vi "Core.vi"() -> (19 "Error Out":errorcluster)   [LabVIEW 2017]
uses:
  <vilib>/Platform/TimedLoop/XDataNode/timing_clust.ctl
  <vilib>/Platform/TimedLoop/XDataNode/nitl_modes.ctl
  <vilib>/Platform/TimedLoop/XDataNode/wakeup.ctl
  <vilib>/Platform/TimedLoop/XDataNode/XDataNode.xnode
  <vilib>/Platform/TimedLoop/XDataNode/XDNodeRunTimeDep.lvlib
panel:
  out "Output Resistance 2":dbl
  in  "Shutdown":bool
  out "Output Resistance":dbl
  # "Core Module DIagnostics"
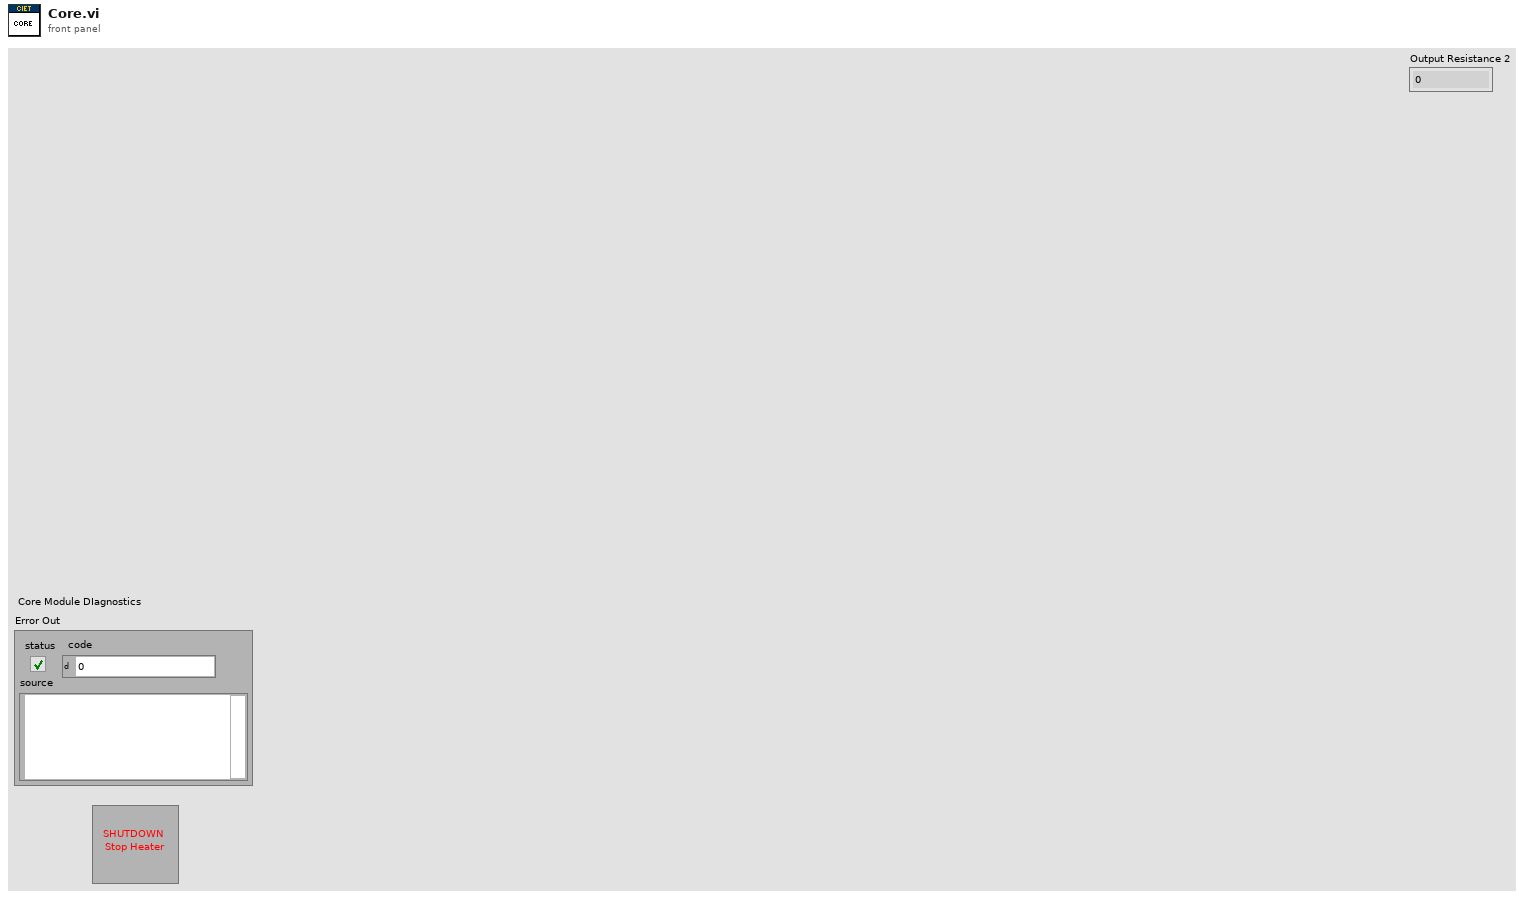
[diagram p1: front panel]
types:
  T1 = typedef "XDNodeRunTimeDep.lvlib/timing_clust.ctl" = cluster{"Expected End [f-1]":u64, "Actual End [f-1]":u64, "Finished Late? [f-1]":bool, "Expected End [i-1]":u64, "Actual End [i-1]":u64, "Finished Late? [i-1]":bool, "Expected Start [i]":u64, "Actual Start [i]":u64, "Expected Start [f]":u64, "Actual Start [f]":u64, "Source Name":string, "Structure Name":string, "Period":i64, "Deadline":i64, "Offset":i64, "Start":i64, "Priority":i32, "Timeout":i32, "Mode":T2, "Wakeup Reason":T3, "Error":errorcluster, "Source Type":string, "Secondary Source Type":string, "Global End Time":u64, "Global Start Time":u64, "Frame Duration":u64, "Iteration Duration":u64, "Assigned CPU":i32, "I/O Scan Engine Mode":u32}
  T2 = typedef "XDNodeRunTimeDep.lvlib/nitl_modes.ctl" = enum32{"No Change", "Process missed periods, maintain original phase", "Discard missed periods, maintain original phase", "Process missed periods, ignore original phase", "Discard missed periods, ignore original phase"}
  T3 = typedef "XDNodeRunTimeDep.lvlib/wakeup.ctl" = enum32{"Normal", "Aborted", "Asynchronous wakeup", "Timing source error", "Timed loop error", "Timeout"}
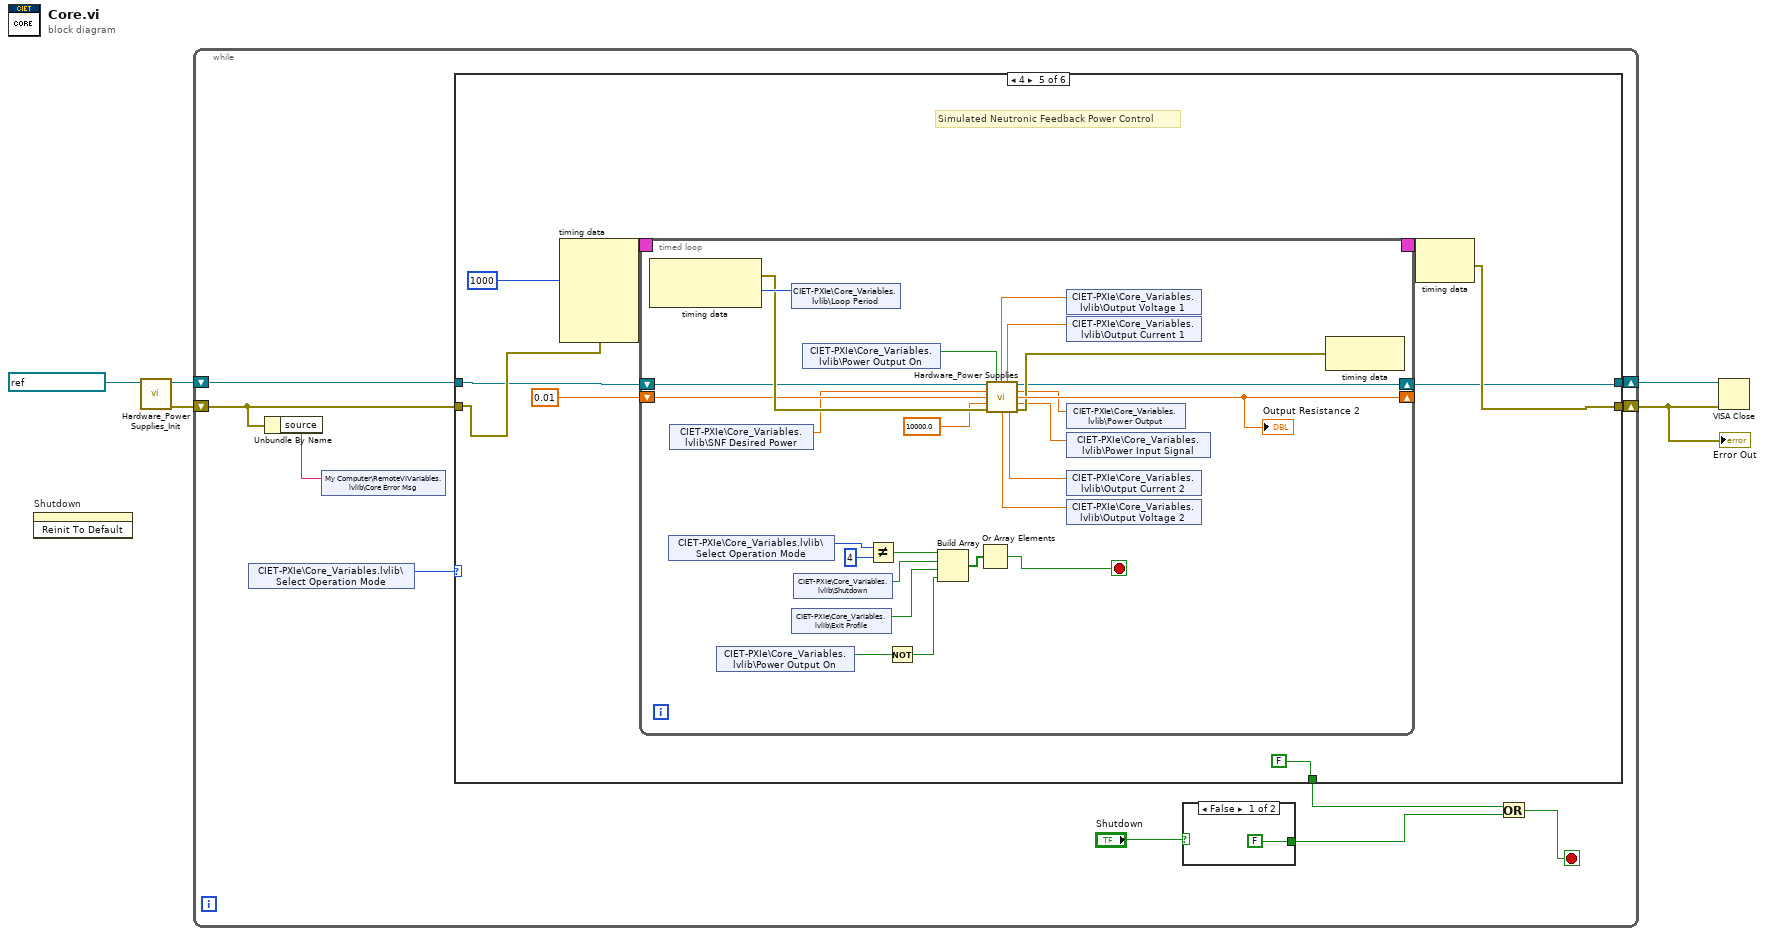
[diagram p0: block diagram]
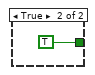
[diagram p2: hidden frame]
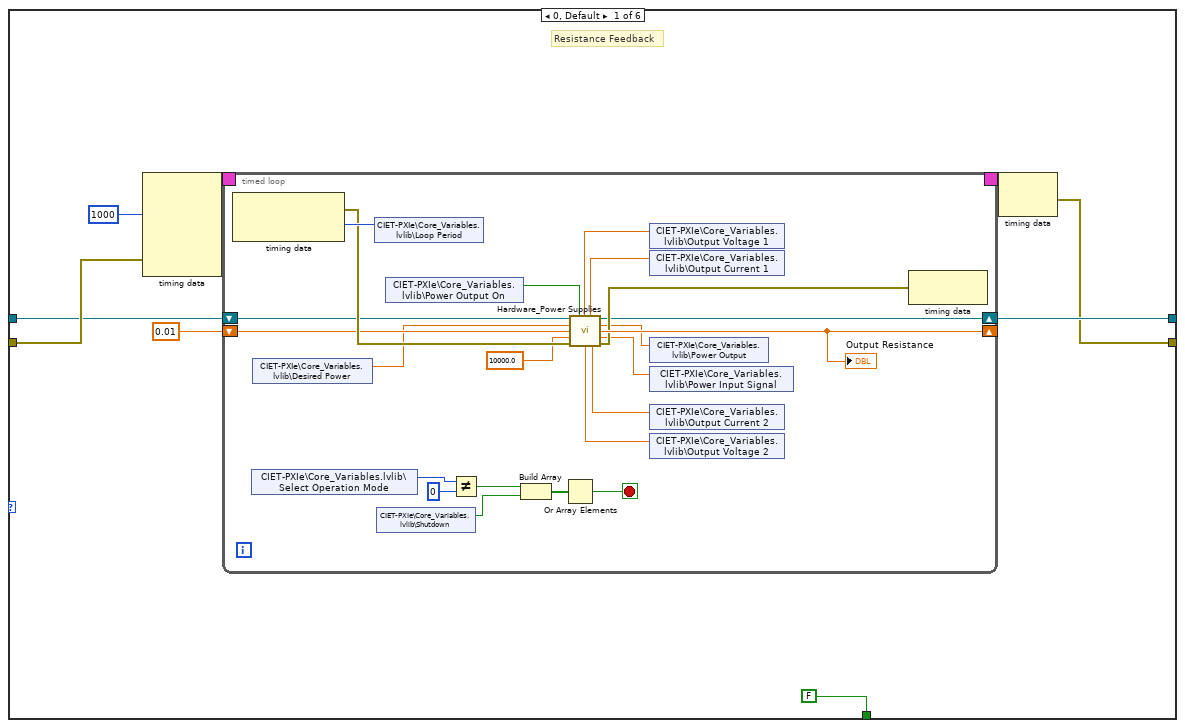
[diagram p3: hidden frame]
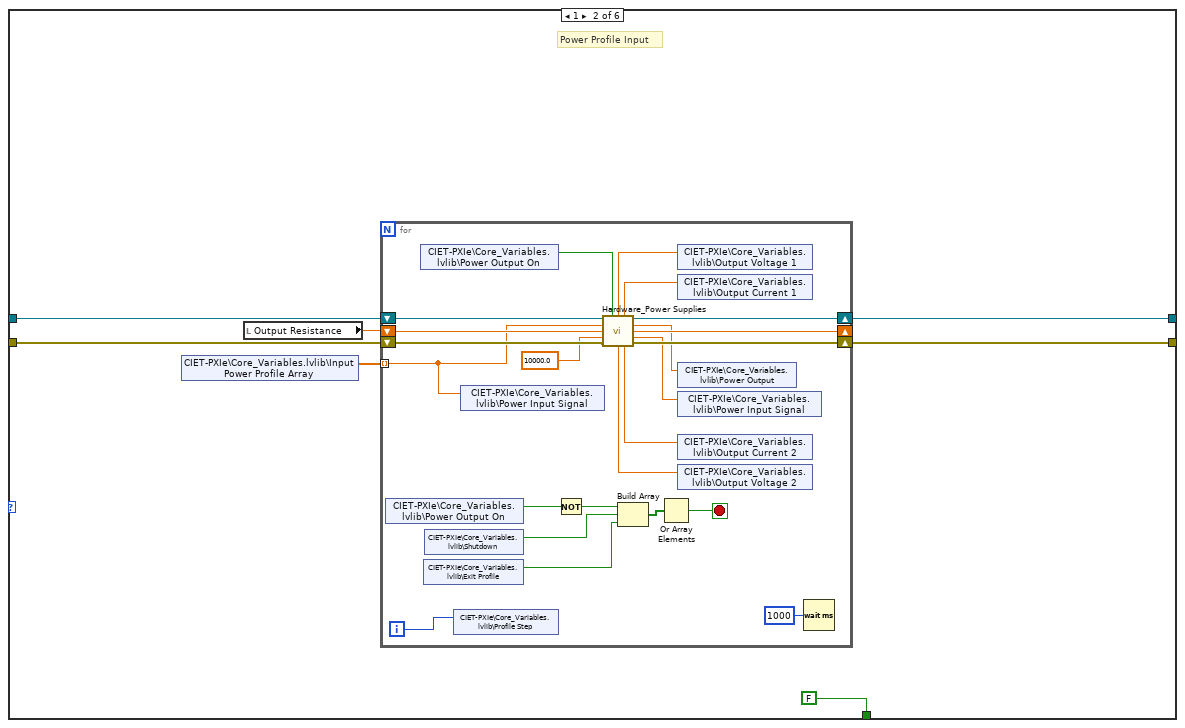
[diagram p4: hidden frame]
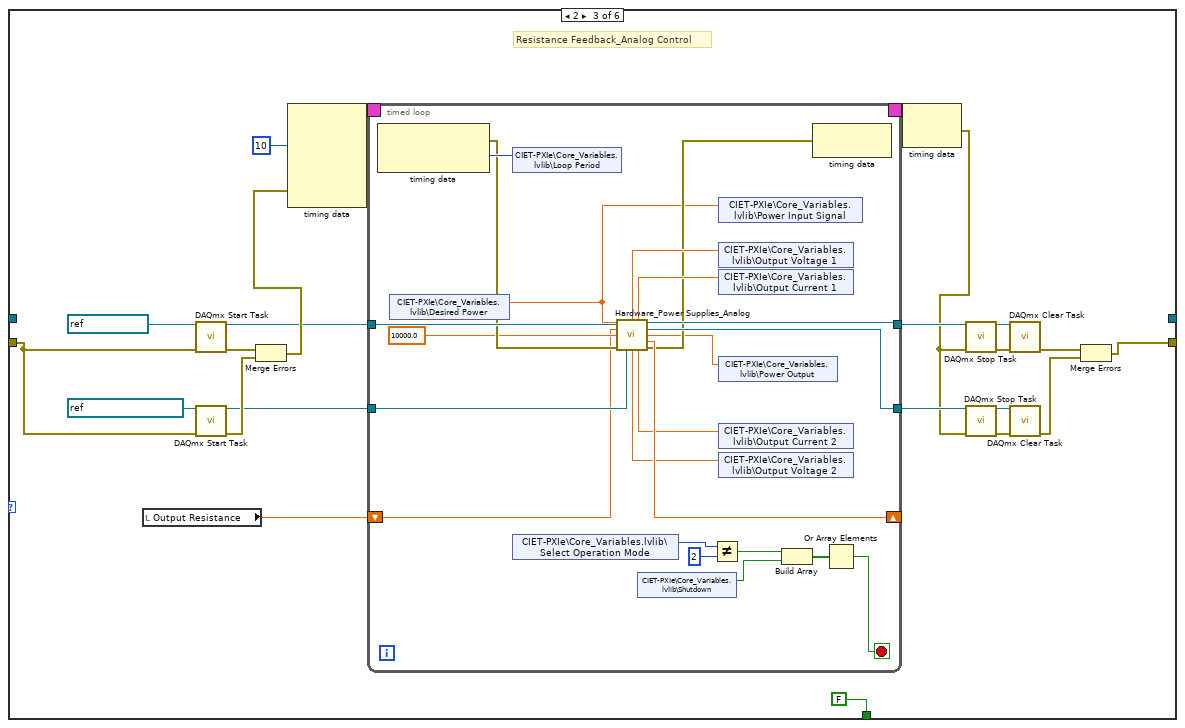
[diagram p5: hidden frame]
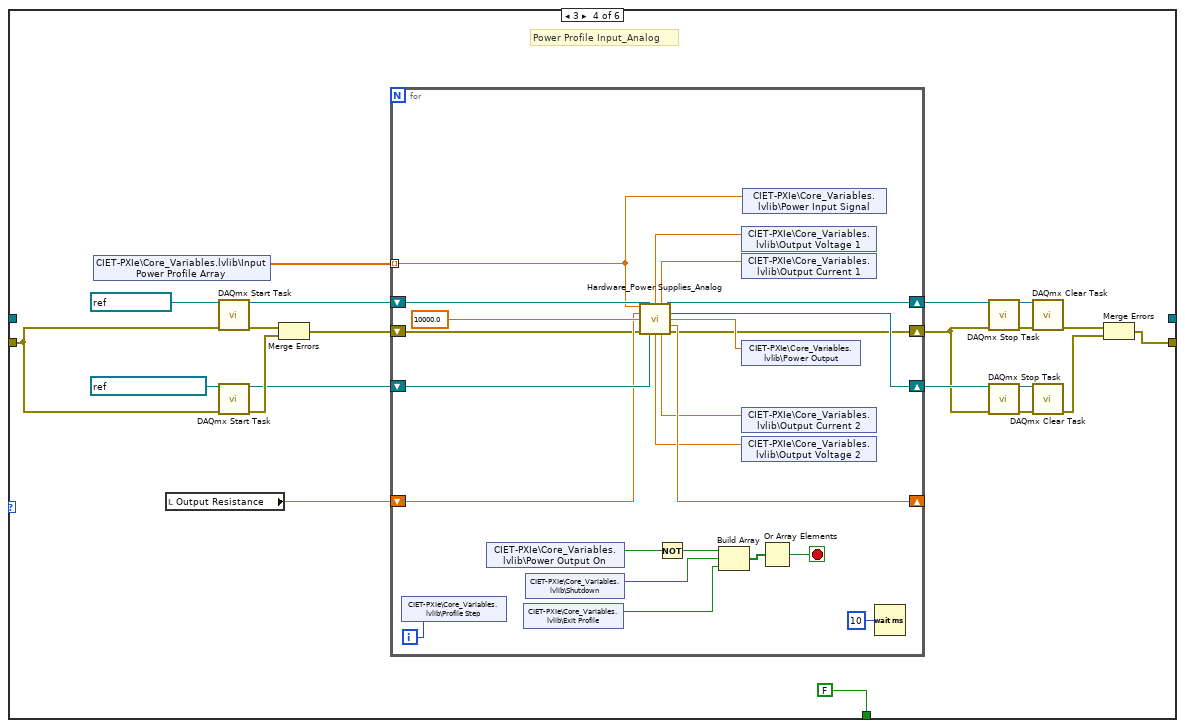
[diagram p6: hidden frame]
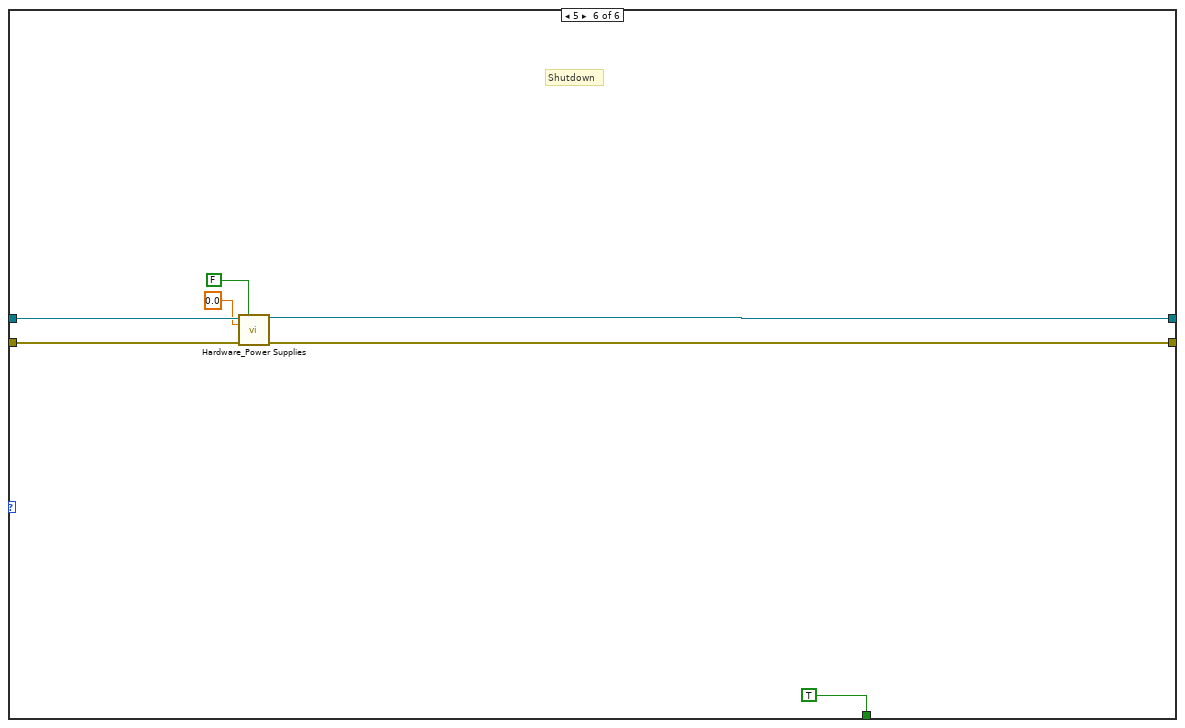
[diagram p7: hidden frame]
diagram:
  n1 = invoke on="Shutdown" class="Bool (strict)" method="Reinit To Default"() -> ()  [unwired: 3 in, 3 out]
  n2 = call "Hardware_Power Supplies_Init.vi"("VISA name"=refnum<visa-resource-name> "PowerSupply") -> ("Error out"=w1:errorcluster, "VISA out"=w2:refnum<visa-resource-name>)  [unwired: 9 in]
  n3 = while {
    shift-right: [w13] -> w4
    shift-left: w1 -> [w7]
    shift-right: [w14] -> w5
    shift-left: w2 -> [w15]
    stop <- w9 stop-if-true
    n4 = shared-variable "CIET-PXIe\\Core_Variables.lvlib\\Select Operation Mode"() -> (w12:u16)  [unwired: 1 in, 1 out]
    n5 = Unbundle By Name(w7) -> ("source"=w6:string)
    n6 = shared-variable "My Computer\\RemoteVIVariables.lvlib\\Core Error Msg"(w6) -> ()  [unwired: 1 in, 1 out]
    n7 = case shown="4" w12 {
      tunnel: w7 -> [w24 w64 w98 w153 w195 w243]
      tunnel: w15 -> [w23 w67 _ _ w194 w242]
      tunnel: [w21 w66 _ _ w193 w241] -> w14
      tunnel: [w20 w63 w103 w152 w196 w240] -> w13
      tunnel: [FALSE ("Shutdown") FALSE ("Shutdown") FALSE ("Shutdown") FALSE ("Shutdown") FALSE ("Shutdown") TRUE ("Shutdown")] -> w11
      frame 0, Default {
        # "Resistance Feedback"
        n8 = node-c288(i64 1000 ("Period"), w24) -> (w26:T1)  [unwired: 3 in]
        n9 = timed-loop {
          timing: w26 -> [_]
          timing-out: [_] -> w25
          shift-right: [w33] -> w21
          shift-left: w23 -> [w40]
          shift-right: [w37] -> _
          shift-left: 0.01 -> [w39]
          stop <- w45 stop-if-true
          n10 = node-c288() -> (w41:errorcluster, w44:i64)  [unwired: 1 in]
          n11 = shared-variable "CIET-PXIe\\Core_Variables.lvlib\\Select Operation Mode"() -> (w43:u16)  [unwired: 1 in, 1 out]
          n12 = shared-variable "CIET-PXIe\\Core_Variables.lvlib\\Desired Power"() -> (w27:dbl)  [unwired: 1 in, 1 out]
          n13 = shared-variable "CIET-PXIe\\Core_Variables.lvlib\\Loop Period"(w44) -> ()  [unwired: 1 in, 1 out]
          n14 = shared-variable "CIET-PXIe\\Core_Variables.lvlib\\Shutdown"() -> (w42:bool)  [unwired: 1 in, 1 out]
          n15 = shared-variable "CIET-PXIe\\Core_Variables.lvlib\\Power Output On"() -> (w32:bool)  [unwired: 1 in, 1 out]
          n16 = Not Equal?(x=w43, y=u16 0) -> (x != y?=w47:bool)
          n17 = Build Array(w47, w42) -> (w46:bool[])
          n18 = Or Array Elements(Boolean array=w46) -> (logical OR=w45:bool)
          n19 = call "Hardware_Power Supplies.vi"("Input VISA"=w40, "Power Output ON"=w32, "Desired Power"=w27, "Input Resistance"=w39, "Maximum Power Limit"=10000.0, "Input Error"=w41) -> ("Output Voltage 1"=w31:dbl, "Output Current 1"=w30:dbl, "Output VISA"=w33:refnum<visa-resource-name>, "Output Power"=w34:dbl, "Output Resistance"=w37:dbl, "Input Power"=w35:dbl, "Output Voltage 2"=w28:dbl, "Output Current 2"=w29:dbl, "Output Error"=w36:errorcluster)  [unwired: 1 in]
          "Output Resistance" <- w37
          n20 = shared-variable "CIET-PXIe\\Core_Variables.lvlib\\Output Voltage 1"(w31) -> ()  [unwired: 1 in, 1 out]
          n21 = shared-variable "CIET-PXIe\\Core_Variables.lvlib\\Output Current 1"(w30) -> ()  [unwired: 1 in, 1 out]
          n22 = shared-variable "CIET-PXIe\\Core_Variables.lvlib\\Power Output"(w34) -> ()  [unwired: 1 in, 1 out]
          n23 = shared-variable "CIET-PXIe\\Core_Variables.lvlib\\Power Input Signal"(w35) -> ()  [unwired: 1 in, 1 out]
          n24 = shared-variable "CIET-PXIe\\Core_Variables.lvlib\\Output Current 2"(w29) -> ()  [unwired: 1 in, 1 out]
          n25 = shared-variable "CIET-PXIe\\Core_Variables.lvlib\\Output Voltage 2"(w28) -> ()  [unwired: 1 in, 1 out]
          n26 = node-c288(w36) -> ()  [unwired: 1 out]
        }
        n27 = node-c288(w25) -> (w20:errorcluster)
      }
      frame 1 {
        # "Power Profile Input"
        n28 = shared-variable "CIET-PXIe\\Core_Variables.lvlib\\Input Power Profile Array"() -> (w61:dbl[])  [unwired: 1 in, 1 out]
        n29 = local read "Output Resistance"() -> (w65:dbl)
        n30 = for {
          shift-right: [w82] -> w66
          shift-left: w67 -> [w83]
          shift-right: [w81] -> w63
          shift-left: w64 -> [w80]
          tunnel: w61 -> [w68] mode=indexing
          shift-right: [w74] -> _
          shift-left: w65 -> [w73]
          i -> [w84]
          stop <- w88 stop-if-true
          n31 = shared-variable "CIET-PXIe\\Core_Variables.lvlib\\Power Output On"() -> (w86:bool)  [unwired: 1 in, 1 out]
          n32 = shared-variable "CIET-PXIe\\Core_Variables.lvlib\\Power Output On"() -> (w79:bool)  [unwired: 1 in, 1 out]
          n33 = shared-variable "CIET-PXIe\\Core_Variables.lvlib\\Exit Profile"() -> (w69:bool)  [unwired: 1 in, 1 out]
          n34 = shared-variable "CIET-PXIe\\Core_Variables.lvlib\\Shutdown"() -> (w85:bool)  [unwired: 1 in, 1 out]
          n35 = shared-variable "CIET-PXIe\\Core_Variables.lvlib\\Profile Step"(w84) -> ()  [unwired: 1 in, 1 out]
          n36 = shared-variable "CIET-PXIe\\Core_Variables.lvlib\\Power Input Signal"(w68) -> ()  [unwired: 1 in, 1 out]
          n37 = Not(x=w86) -> (.not. x?=w87:bool)
          n38 = call "Hardware_Power Supplies.vi"("Input VISA"=w83, "Power Output ON"=w79, "Desired Power"=w68, "Input Resistance"=w73, "Maximum Power Limit"=10000.0, "Input Error"=w80) -> ("Output Voltage 1"=w78:dbl, "Output Current 1"=w77:dbl, "Output VISA"=w82:refnum<visa-resource-name>, "Output Power"=w71:dbl, "Output Resistance"=w74:dbl, "Input Power"=w70:dbl, "Output Voltage 2"=w76:dbl, "Output Current 2"=w75:dbl, "Output Error"=w81:errorcluster)  [unwired: 1 in]
          n39 = Build Array(w87, w85, w69) -> (w90:bool[])
          n40 = Or Array Elements(Boolean array=w90) -> (logical OR=w88:bool)
          n41 = shared-variable "CIET-PXIe\\Core_Variables.lvlib\\Output Voltage 1"(w78) -> ()  [unwired: 1 in, 1 out]
          n42 = shared-variable "CIET-PXIe\\Core_Variables.lvlib\\Output Current 1"(w77) -> ()  [unwired: 1 in, 1 out]
          n43 = shared-variable "CIET-PXIe\\Core_Variables.lvlib\\Power Output"(w71) -> ()  [unwired: 1 in, 1 out]
          n44 = shared-variable "CIET-PXIe\\Core_Variables.lvlib\\Power Input Signal"(w70) -> ()  [unwired: 1 in, 1 out]
          n45 = shared-variable "CIET-PXIe\\Core_Variables.lvlib\\Output Current 2"(w75) -> ()  [unwired: 1 in, 1 out]
          n46 = shared-variable "CIET-PXIe\\Core_Variables.lvlib\\Output Voltage 2"(w76) -> ()  [unwired: 1 in, 1 out]
          n47 = Wait (ms)(milliseconds to wait=u32 1000) -> ()  [unwired: 1 out]
        }
      }
      frame 2 {
        # "Resistance Feedback_Analog Control"
        n48 = local read "Output Resistance"() -> (w95:dbl)
        n49 = call <vilib>:"DAQmx Start Task.vi"("task/channels in"=refnum<k21> "PowerOut", "error in"=w98) -> ("task out"=w97:refnum<k21>, "error out"=w113:errorcluster)  [unwired: 12 in]
        n50 = call <vilib>:"DAQmx Start Task.vi"("task/channels in"=refnum<k21> "PowerMonitor_V", "error in"=w98) -> ("task out"=w96:refnum<k21>, "error out"=w112:errorcluster)  [unwired: 12 in]
        n51 = Merge Errors(w113, w112) -> (w99:errorcluster)
        n52 = node-c288(i64 10 ("Period"), w99) -> (w102:T1)  [unwired: 3 in]
        n53 = timed-loop {
          timing: w102 -> [_]
          timing-out: [_] -> w101
          shift-right: [w129] -> _
          shift-left: w95 -> [w130]
          tunnel: w97 -> [w134]
          tunnel: [w128] -> w94
          tunnel: w96 -> [w133]
          tunnel: [w127] -> w93
          stop <- w115 stop-if-true
          n54 = node-c288() -> (w132:errorcluster, w135:i64)  [unwired: 1 in]
          n55 = shared-variable "CIET-PXIe\\Core_Variables.lvlib\\Desired Power"() -> (w114:dbl)  [unwired: 1 in, 1 out]
          n56 = shared-variable "CIET-PXIe\\Core_Variables.lvlib\\Loop Period"(w135) -> ()  [unwired: 1 in, 1 out]
          n57 = shared-variable "CIET-PXIe\\Core_Variables.lvlib\\Select Operation Mode"() -> (w117:u16)  [unwired: 1 in, 1 out]
          n58 = call "Hardware_Power Supplies_Analog.vi"("Desired Power"=w114, "Task In_1"=w134, "Input Resistance"=w130, "Maximum Power Limit"=10000.0, "Error In"=w132, "Task In_2"=w133) -> ("Output Voltage 1"=w126:dbl, "Output Current 1"=w125:dbl, "Task Out_1"=w128:refnum<k21>, "Task Out_2"=w127:refnum<k21>, "Output Power"=w121:dbl, "Output Resistance"=w129:dbl, "Output Voltage 2"=w124:dbl, "Output Current 2"=w123:dbl, "Error Out"=w122:errorcluster)  [unwired: 1 in]
          n59 = shared-variable "CIET-PXIe\\Core_Variables.lvlib\\Shutdown"() -> (w116:bool)  [unwired: 1 in, 1 out]
          n60 = Not Equal?(x=w117, y=u16 2) -> (x != y?=w119:bool)
          n61 = shared-variable "CIET-PXIe\\Core_Variables.lvlib\\Power Input Signal"(w114) -> ()  [unwired: 1 in, 1 out]
          n62 = shared-variable "CIET-PXIe\\Core_Variables.lvlib\\Output Voltage 1"(w126) -> ()  [unwired: 1 in, 1 out]
          n63 = shared-variable "CIET-PXIe\\Core_Variables.lvlib\\Output Current 1"(w125) -> ()  [unwired: 1 in, 1 out]
          n64 = shared-variable "CIET-PXIe\\Core_Variables.lvlib\\Power Output"(w121) -> ()  [unwired: 1 in, 1 out]
          n65 = shared-variable "CIET-PXIe\\Core_Variables.lvlib\\Output Current 2"(w123) -> ()  [unwired: 1 in, 1 out]
          n66 = shared-variable "CIET-PXIe\\Core_Variables.lvlib\\Output Voltage 2"(w124) -> ()  [unwired: 1 in, 1 out]
          n67 = Build Array(w119, w116) -> (w118:bool[])
          n68 = node-c288(w122) -> ()  [unwired: 1 out]
          n69 = Or Array Elements(Boolean array=w118) -> (logical OR=w115:bool)
        }
        n70 = node-c288(w101) -> (w91:errorcluster)
        n71 = call <vilib>:"DAQmx Stop Task.vi"("task/channels in"=w94, "error in"=w91) -> ("task out"=w109:refnum<k21>, "error out"=w108:errorcluster)  [unwired: 12 in]
        n72 = call <vilib>:"DAQmx Stop Task.vi"("task/channels in"=w93, "error in"=w91) -> ("task out"=w107:refnum<k21>, "error out"=w106:errorcluster)  [unwired: 12 in]
        n73 = call <vilib>:"DAQmx Clear Task.vi"("task in"=w109, "error in"=w108) -> ("error out"=w105:errorcluster)  [unwired: 13 in]
        n74 = call <vilib>:"DAQmx Clear Task.vi"("task in"=w107, "error in"=w106) -> ("error out"=w104:errorcluster)  [unwired: 13 in]
        n75 = Merge Errors(w105, w104) -> (w103:errorcluster)
      }
      frame 3 {
        # "Power Profile Input_Analog"
        n76 = shared-variable "CIET-PXIe\\Core_Variables.lvlib\\Input Power Profile Array"() -> (w149:dbl[])  [unwired: 1 in, 1 out]
        n77 = local read "Output Resistance"() -> (w156:dbl)
        n78 = call <vilib>:"DAQmx Start Task.vi"("task/channels in"=refnum<k21> "PowerOut", "error in"=w153) -> ("task out"=w158:refnum<k21>, "error out"=w168:errorcluster)  [unwired: 12 in]
        n79 = call <vilib>:"DAQmx Start Task.vi"("task/channels in"=refnum<k21> "PowerMonitor_V", "error in"=w153) -> ("task out"=w157:refnum<k21>, "error out"=w167:errorcluster)  [unwired: 12 in]
        n80 = Merge Errors(w168, w167) -> (w151:errorcluster)
        n81 = for {
          shift-right: [w187] -> _
          shift-left: w156 -> [w188]
          shift-right: [w186] -> w155
          shift-left: w158 -> [w191]
          shift-right: [w185] -> w154
          shift-left: w157 -> [w190]
          shift-right: [w178] -> w150
          shift-left: w151 -> [w179]
          tunnel: w149 -> [w169] mode=indexing
          i -> [w173]
          stop <- w172 stop-if-true
          n82 = shared-variable "CIET-PXIe\\Core_Variables.lvlib\\Profile Step"(w173) -> ()  [unwired: 1 in, 1 out]
          n83 = shared-variable "CIET-PXIe\\Core_Variables.lvlib\\Power Output On"() -> (w175:bool)  [unwired: 1 in, 1 out]
          n84 = shared-variable "CIET-PXIe\\Core_Variables.lvlib\\Exit Profile"() -> (w170:bool)  [unwired: 1 in, 1 out]
          n85 = shared-variable "CIET-PXIe\\Core_Variables.lvlib\\Shutdown"() -> (w174:bool)  [unwired: 1 in, 1 out]
          n86 = call "Hardware_Power Supplies_Analog.vi"("Desired Power"=w169, "Task In_1"=w191, "Input Resistance"=w188, "Maximum Power Limit"=10000.0, "Error In"=w179, "Task In_2"=w190) -> ("Output Voltage 1"=w184:dbl, "Output Current 1"=w183:dbl, "Task Out_1"=w186:refnum<k21>, "Task Out_2"=w185:refnum<k21>, "Output Power"=w180:dbl, "Output Resistance"=w187:dbl, "Output Voltage 2"=w182:dbl, "Output Current 2"=w181:dbl, "Error Out"=w178:errorcluster)  [unwired: 1 in]
          n87 = Not(x=w175) -> (.not. x?=w176:bool)
          n88 = Build Array(w176, w174, w170) -> (w177:bool[])
          n89 = shared-variable "CIET-PXIe\\Core_Variables.lvlib\\Output Voltage 1"(w184) -> ()  [unwired: 1 in, 1 out]
          n90 = shared-variable "CIET-PXIe\\Core_Variables.lvlib\\Output Current 1"(w183) -> ()  [unwired: 1 in, 1 out]
          n91 = shared-variable "CIET-PXIe\\Core_Variables.lvlib\\Power Output"(w180) -> ()  [unwired: 1 in, 1 out]
          n92 = shared-variable "CIET-PXIe\\Core_Variables.lvlib\\Output Current 2"(w181) -> ()  [unwired: 1 in, 1 out]
          n93 = shared-variable "CIET-PXIe\\Core_Variables.lvlib\\Output Voltage 2"(w182) -> ()  [unwired: 1 in, 1 out]
          n94 = shared-variable "CIET-PXIe\\Core_Variables.lvlib\\Power Input Signal"(w169) -> ()  [unwired: 1 in, 1 out]
          n95 = Or Array Elements(Boolean array=w177) -> (logical OR=w172:bool)
          n96 = Wait (ms)(milliseconds to wait=u32 10) -> ()  [unwired: 1 out]
        }
        n97 = call <vilib>:"DAQmx Stop Task.vi"("task/channels in"=w155, "error in"=w150) -> ("task out"=w164:refnum<k21>, "error out"=w163:errorcluster)  [unwired: 12 in]
        n98 = call <vilib>:"DAQmx Stop Task.vi"("task/channels in"=w154, "error in"=w150) -> ("task out"=w162:refnum<k21>, "error out"=w161:errorcluster)  [unwired: 12 in]
        n99 = call <vilib>:"DAQmx Clear Task.vi"("task in"=w164, "error in"=w163) -> ("error out"=w160:errorcluster)  [unwired: 13 in]
        n100 = call <vilib>:"DAQmx Clear Task.vi"("task in"=w162, "error in"=w161) -> ("error out"=w159:errorcluster)  [unwired: 13 in]
        n101 = Merge Errors(w160, w159) -> (w152:errorcluster)
      }
      frame 4 {
        # "Simulated Neutronic Feedback Power Control"
        n102 = node-c288(i64 1000 ("Period"), w195) -> (w200:T1)  [unwired: 3 in]
        n103 = timed-loop {
          timing: w200 -> [_]
          timing-out: [_] -> w199
          shift-right: [w210] -> w193
          shift-left: w194 -> [w217]
          shift-right: [w214] -> _
          shift-left: 0.01 -> [w216]
          stop <- w222 stop-if-true
          n104 = node-c288() -> (w218:errorcluster, w221:i64)  [unwired: 1 in]
          n105 = shared-variable "CIET-PXIe\\Core_Variables.lvlib\\Select Operation Mode"() -> (w220:u16)  [unwired: 1 in, 1 out]
          n106 = shared-variable "CIET-PXIe\\Core_Variables.lvlib\\SNF Desired Power"() -> (w204:dbl)  [unwired: 1 in, 1 out]
          n107 = shared-variable "CIET-PXIe\\Core_Variables.lvlib\\Power Output On"() -> (w203:bool)  [unwired: 1 in, 1 out]
          n108 = shared-variable "CIET-PXIe\\Core_Variables.lvlib\\Loop Period"(w221) -> ()  [unwired: 1 in, 1 out]
          n109 = shared-variable "CIET-PXIe\\Core_Variables.lvlib\\Exit Profile"() -> (w202:bool)  [unwired: 1 in, 1 out]
          n110 = shared-variable "CIET-PXIe\\Core_Variables.lvlib\\Shutdown"() -> (w219:bool)  [unwired: 1 in, 1 out]
          n111 = shared-variable "CIET-PXIe\\Core_Variables.lvlib\\Power Output On"() -> (w209:bool)  [unwired: 1 in, 1 out]
          n112 = Not Equal?(x=w220, y=u16 4) -> (x != y?=w224:bool)
          n113 = Not(x=w203) -> (.not. x?=w201:bool)
          n114 = Build Array(w224, w219, w202, w201) -> (w223:bool[])
          n115 = Or Array Elements(Boolean array=w223) -> (logical OR=w222:bool)
          n116 = call "Hardware_Power Supplies.vi"("Input VISA"=w217, "Power Output ON"=w209, "Desired Power"=w204, "Input Resistance"=w216, "Maximum Power Limit"=10000.0, "Input Error"=w218) -> ("Output Voltage 1"=w208:dbl, "Output Current 1"=w207:dbl, "Output VISA"=w210:refnum<visa-resource-name>, "Output Power"=w211:dbl, "Output Resistance"=w214:dbl, "Input Power"=w212:dbl, "Output Voltage 2"=w205:dbl, "Output Current 2"=w206:dbl, "Output Error"=w213:errorcluster)  [unwired: 1 in]
          "Output Resistance 2" <- w214
          n117 = shared-variable "CIET-PXIe\\Core_Variables.lvlib\\Output Voltage 1"(w208) -> ()  [unwired: 1 in, 1 out]
          n118 = shared-variable "CIET-PXIe\\Core_Variables.lvlib\\Output Current 1"(w207) -> ()  [unwired: 1 in, 1 out]
          n119 = shared-variable "CIET-PXIe\\Core_Variables.lvlib\\Power Output"(w211) -> ()  [unwired: 1 in, 1 out]
          n120 = shared-variable "CIET-PXIe\\Core_Variables.lvlib\\Power Input Signal"(w212) -> ()  [unwired: 1 in, 1 out]
          n121 = shared-variable "CIET-PXIe\\Core_Variables.lvlib\\Output Current 2"(w206) -> ()  [unwired: 1 in, 1 out]
          n122 = shared-variable "CIET-PXIe\\Core_Variables.lvlib\\Output Voltage 2"(w205) -> ()  [unwired: 1 in, 1 out]
          n123 = node-c288(w213) -> ()  [unwired: 1 out]
        }
        n124 = node-c288(w199) -> (w196:errorcluster)
      }
      frame 5 {
        # "Shutdown"
        n125 = call "Hardware_Power Supplies.vi"("Input VISA"=w242, "Power Output ON"=FALSE, "Desired Power"=0.0, "Input Error"=w243) -> ("Output VISA"=w241:refnum<visa-resource-name>, "Output Error"=w240:errorcluster)  [unwired: 3 in, 7 out]
      }
    }
    n126 = case shown="False" "Shutdown" {
      tunnel: [FALSE ("Shutdown") TRUE ("Shutdown")] -> w10
      frame False {
      }
      frame True {
      }
    }
    n127 = Or(x=w11, y=w10) -> (x .or. y?=w9:bool)
  }
  "Error Out" <- w4
  n128 = VISA Close(VISA resource name=w5, error in (no error)=w4) -> ()  [unwired: 1 out]
